vi "Write Data.vi"(8 "error in (no error)":errorcluster, 11 "TDMS Data Logger Actor in":refnum<class "TDMS Data Logger Actor.lvclass">) -> (0 "error out":errorcluster, 3 "TDMS Data Logger Actor out":refnum<class "TDMS Data Logger Actor.lvclass">)   [LabVIEW 2024, in "TDMS Data Logger Actor.lvlib" / "TDMS Data Logger Actor.lvclass"]
uses:
  TDMS Data Logger Actor.lvclass
  TDMS Data Logger Actor.lvclass/TDMS Data Logger Actor.ctl
  Logging Data Interface/Logging Data Interface/Logging Data Interface.lvclass
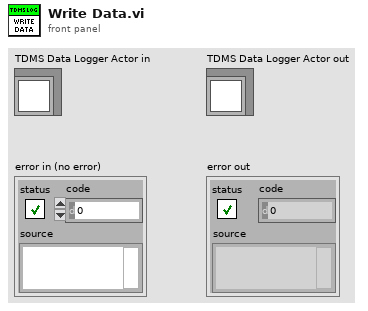
[diagram p1: front panel]
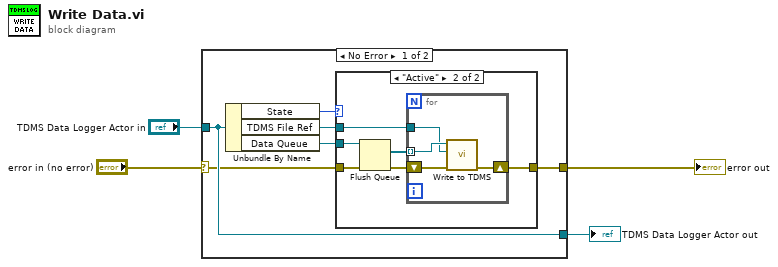
[diagram p0: block diagram]
diagram:
  n1 = case shown="No Error" "error in (no error)" {
    selector: "error in (no error)" -> [w7 w23]
    tunnel: [w6 w23] -> w3
    tunnel: [w10 w22] -> w1
    tunnel: "TDMS Data Logger Actor in" -> [w10 w22]
    frame No Error {
      n2 = Unbundle By Name(w10) -> ("State"=w9:enum16{"Idle", "Active", "Paused"}, "TDMS File Ref"=w8:refnum<k34>, "Data Queue"=w5:refnum<queue>)
      n3 = case shown="\"Active\"" w9 {
        tunnel: w8 -> [_ w12]
        tunnel: w7 -> [w11 w16]
        tunnel: [w11 w17] -> w6
        tunnel: w5 -> [_ w13]
        frame "Idle", "Paused" {
        }
        frame "Active" {
          n4 = Flush Queue(queue=w13, error in (no error)=w16) -> (remaining elements=w14:refnum<class "Logging Data Interface.lvclass">[], error out=w15:errorcluster)  [unwired: 1 out]
          n5 = for {
            shift-right: [w18] -> w17
            shift-left: w15 -> [w19]
            tunnel: w14 -> [w21] mode=indexing
            tunnel: w12 -> [w20]
            n6 = call-dynamic "Write to TDMS.vi"("error in (no error)"=w19, "TDMS File Ref"=w20, "Logging Data Interface in"=w21) -> ("error out"=w18:errorcluster)  [unwired: 8 in]
          }
        }
      }
    }
    frame Error {
    }
  }
  "error out" <- w3
  "TDMS Data Logger Actor out" <- w1
